vi "NISE.local.Reset Devices.vi"(0 "SLSC Local in":refnum<class "SLSC Interface.lvclass">, 5 "devices":refnum<k21>="$DefaultDevices", 11 "error in (no error)":errorcluster) -> (4 "SLSC Local out":refnum<class "SLSC Interface.lvclass">, 15 "error out":errorcluster)   [LabVIEW 2016, in "SLSC Interface.lvclass"]
uses:
  SLSC Interface Class/SLSC Interface.lvclass
  SLSC Interface Class/NISE.Read session.vi
  SLSC Interface Class/NISE.Write session.vi
  <vilib>/SLSC/SLSC.lvlib
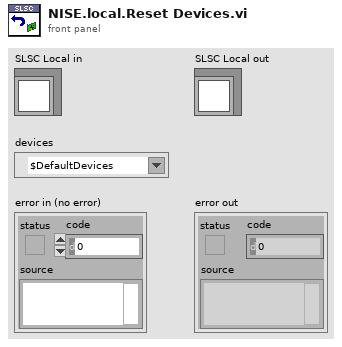
[diagram p1: front panel]
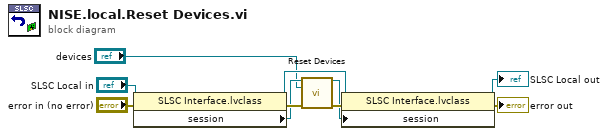
[diagram p0: block diagram]
diagram:
  n1 = property class="SLSC Interface.lvclass"(reference="SLSC Local in", error in="error in (no error)") -> (reference out=w7:refnum<class "SLSC Interface.lvclass">, error out=w9:errorcluster, "session"=w5:refnum<k21>)
  n2 = call <vilib>:"Reset Devices.vi"("session in"=w5, "devices"="devices", "error in (no error)"=w9) -> ("session out"=w4:refnum<k21>, "error out"=w8:errorcluster)  [unwired: 11 in]
  n3 = property class="SLSC Interface.lvclass"(reference=w7, error in=w8, "session"=w4) -> (reference out=→"SLSC Local out":refnum<class "SLSC Interface.lvclass">, error out=→"error out":errorcluster)
